vi "apply key value pairs.vi"(8 "error in":errorcluster, 9 "values":string[](array[string]), 10 "keys":string[](array[string]), 11 "fixed channel runtime in":refnum<class "ScaleAndLimitModule runtime.lvclass">) -> (0 "error out":errorcluster, 3 "fixed channel runtime out":refnum<class "ScaleAndLimitModule runtime.lvclass">)   [LabVIEW 2017, in "ScaleAndLimitModule runtime.lvclass"]
uses:
  ScaleAndLimitModule runtime.lvclass
  ScaleAndLimitModule runtime.lvclass/ScaleAndLimitModule runtime.ctl
  <vilib>/NI/PowerElectronicsControl/ScaleAndLimit/Interface/Configuration.ctl
  <vilib>/NI/PowerElectronicsControl/ScaleAndLimit/Interface/ScaleAndLimitInterface.lvlib
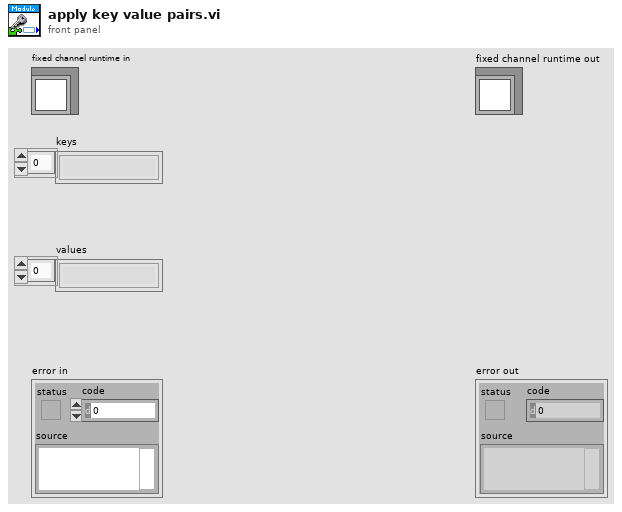
[diagram p1: front panel]
types:
  T1 = typedef "ScaleAndLimitInterface.lvlib/Configuration.ctl" = cluster{"Name":string, "M":dbl, "B":i16, "HighLimit":dbl, "LowLimit":dbl, "LimitsEnabled":bool}
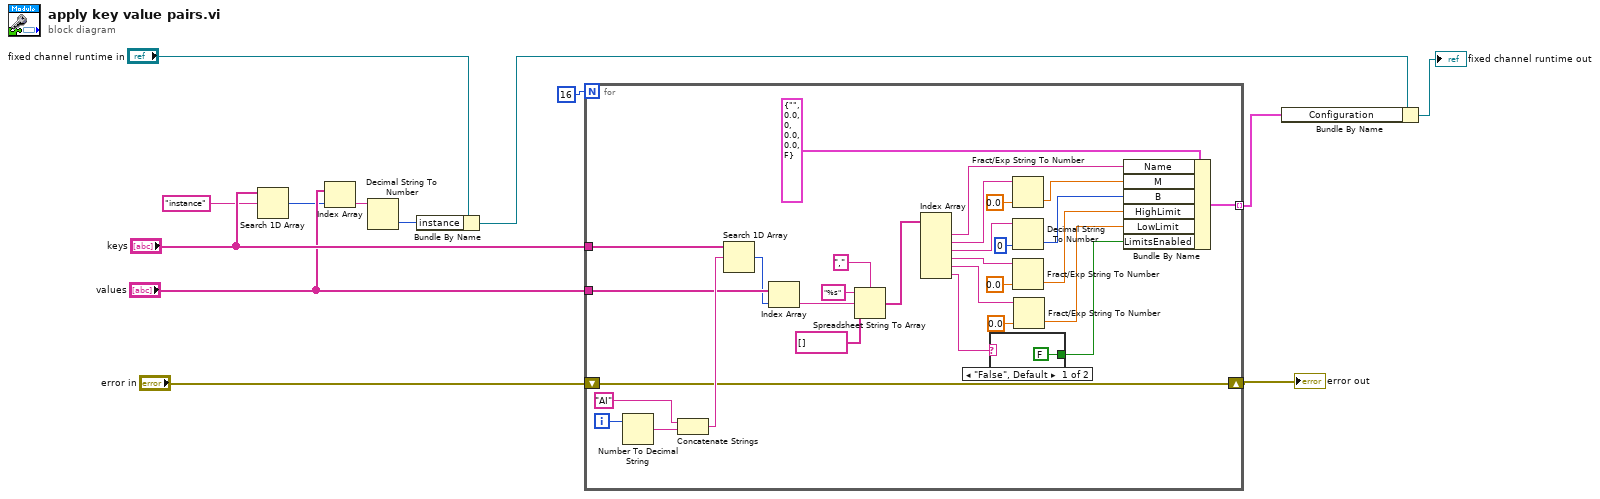
[diagram p0: block diagram]
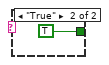
[diagram p2: hidden frame]
diagram:
  n1 = Search 1D Array(1D array="keys", element="instance") -> (index of element=w5:i32)  [unwired: 1 in]
  n2 = Index Array(array="values", index=w5) -> (element=w4:string)
  n3 = Decimal String To Number(string=w4) -> (number=w3:i32)  [unwired: 2 in, 1 out]
  n4 = Bundle By Name(cluster="fixed channel runtime in", "instance"=w3) -> (w1:refnum<class "ScaleAndLimitModule runtime.lvclass">)
  n5 = for {
    N: 16 -> [_]
    tunnel: "keys" -> [w40]
    tunnel: "values" -> [w38]
    shift-right: [w32] -> w11
    shift-left: "error in" -> [w32]
    tunnel: [w15] -> w10 mode=indexing
    i -> [w43]
    n6 = Number To Decimal String(number=w43) -> (decimal integer string=w42:string)  [unwired: 1 in]
    n7 = Concatenate Strings("AI", w42) -> (w39:string)
    n8 = Search 1D Array(1D array=w40, element=w39) -> (index of element=w37:i32)  [unwired: 1 in]
    n9 = Index Array(array=w38, index=w37) -> (element=w36:string)
    n10 = Spreadsheet String To Array(delimiter (Tab)=",", format string="%s", spreadsheet string=w36, array type (2D Dbl)=string[] []) -> (array=w33:string[])
    n11 = Index Array(array=w33) -> (element #1=w30:string, element #2=w29:string, element #3=w26:string, element #4=w21:string, element #5=w20:string, element #6=w17:string)  [unwired: 6 in]
    n12 = case shown="\"False\", Default" w17 {
      tunnel: [FALSE TRUE] -> w16
      frame "False", Default {
      }
      frame "True" {
      }
    }
    n13 = Fract/Exp String To Number(string=w29, default (0 dbl)=sgl 0.0 ("default (0 DBL)")) -> (number=w27:sgl)  [unwired: 2 in, 1 out]
    n14 = Decimal String To Number(string=w26, default (0L)=i16 0 ("B")) -> (number=w24:i16)  [unwired: 1 in, 1 out]
    n15 = Fract/Exp String To Number(string=w21, default (0 dbl)=sgl 0.0 ("default (0 DBL)")) -> (number=w19:sgl)  [unwired: 2 in, 1 out]
    n16 = Fract/Exp String To Number(string=w20, default (0 dbl)=sgl 0.0 ("default (0 DBL)")) -> (number=w18:sgl)  [unwired: 2 in, 1 out]
    n17 = Bundle By Name(cluster=T1 {"Name"="", "M"=0.0, "B"=0, "HighLimit"=0.0, "LowLimit"=0.0, "LimitsEnabled"=FALSE} ("Configuration"), "Name"=w30, "M"=w27, "B"=w24, "HighLimit"=w19, "LowLimit"=w18, "LimitsEnabled"=w16) -> (w15:T1)
  }
  "error out" <- w11
  n18 = Bundle By Name(cluster=w1, "Configuration"=w10) -> (→"fixed channel runtime out":refnum<class "ScaleAndLimitModule runtime.lvclass">)
